vi "log analysis_gps.vi"() -> ()   [LabVIEW 2019] (continued)
-2.475798603,298.940458629,0.4409,0.2946,0.5535,0.1135,0.0926,0.0773,0.0981,0.1029,4.8962,0f000001,0*a1f88c2d\n\t", "INSPVAXA,USB3,0,45.5,FINESTEERING,2107,282909.600,02000000,471d,15824;INS_ALIGNMENT_COMPLETE,INS_RTKFIXED,37.37090578020,126.72380341402,9.0005,22.3000,0.2042,-0.2452,-0.0267,-0.096054371,-2.657817318,299.053399996,0.4409,0.2946,0.5535,0.1135,0.0926,0.0773,0.0981,0.1029,4.8962,0f000001,0*97d4220e\n\t", "INSPVAXA,USB3,0,44.5,FINESTEERING,2107,282910.100,02000000,471d,15824;INS_ALIGNMENT_COMPLETE,INS_RTKFIXED,37.37090649384,126.72380213526,8.9945,22.3000,0.1796,-0.2032,-0.0123,-0.081156055,-2.596786574,299.082136119,0.4412,0.2947,0.5535,0.1135,0.0926,0.0773,0.0981,0.1029,4.8970,0f000001,0*70e9c9df\n\t", "INSPVAXA,USB3,0,44.5,FINESTEERING,2107,282910.600,02000000,471d,15824;INS_ALIGNMENT_COMPLETE,INS_RTKFIXED,37.37090728426,126.72380074897,8.9873,22.3000,0.2078,-0.2346,-0.0218,0.045801771,-2.674891598,299.142927174,0.4412,0.2947,0.5535,0.1135,0.0926,0.0773,0.0981,0.1029,4.8970,0f000001,0*500925c1\n\t", "INSPVAXA,USB3,0,45.5,FINESTEERING,2107,282911.100,02000000,471d,15824;INS_ALIGNMENT_COMPLETE,INS_RTKFIXED,37.37090803309,126.72379945819,8.9800,22.3000,0.1796,-0.1956,-0.0242,0.023894528,-2.705451433,299.250076985,0.4415,0.2948,0.5535,0.1135,0.0925,0.0773,0.0981,0.1029,4.8973,0f000001,0*fcb889be\n\t", "INSPVAXA,USB3,0,45.5,FINESTEERING,2107,282911.600,02000000,471d,15824;INS_ALIGNMENT_COMPLETE,INS_RTKFIXED,37.37090882517,126.72379803977,8.9729,22.3000,0.1992,-0.2347,-0.0122,-0.052701655,-2.537774269,299.314444801,0.4415,0.2948,0.5535,0.1135,0.0925,0.0773,0.0981,0.1029,4.8973,0f000001,0*f806d9f3\n\t", "INSPVAXA,USB3,0,49.0,FINESTEERING,2107,282912.100,02000000,471d,15824;INS_ALIGNMENT_COMPLETE,INS_RTKFIXED,37.37090954144,126.72379680635,8.9662,22.3000,0.2005,-0.2326,-0.0241,-0.125797305,-2.436851943,299.381095140,0.4412,0.2948,0.5534,0.1134,0.0926,0.0773,0.0980,0.1029,4.8978,0f000001,0*e5b9f40a\n\t", "INSPVAXA,USB3,0,49.0,FINESTEERING,2107,282912.600,02000000,471d,15824;INS_ALIGNMENT_COMPLETE,INS_RTKFIXED,37.37091031837,126.72379541279,8.9597,22.3000,0.1852,-0.2068,-0.0204,-0.071142448,-2.486574172,299.492569727,0.4412,0.2948,0.5534,0.1134,0.0926,0.0773,0.0980,0.1029,4.8978,0f000001,0*cac4ba0d\n\t", "INSPVAXA,USB3,0,49.5,FINESTEERING,2107,282913.100,02000000,471d,15824;INS_ALIGNMENT_COMPLETE,INS_RTKFIXED,37.37091108524,126.72379405931,8.9519,22.3000,0.1888,-0.2272,-0.0247,-0.028725670,-2.337365397,299.552597059,0.4407,0.2948,0.5532,0.1133,0.0925,0.0773,0.0980,0.1028,4.8983,0f000001,0*e96bcee1\n\t", "INSPVAXA,USB3,0,49.5,FINESTEERING,2107,282913.600,02000000,471d,15824;INS_ALIGNMENT_COMPLETE,INS_RTKFIXED,37.37091181929,126.72379275953,8.9460,22.3000,0.2010,-0.2341,-0.0266,0.089811982,-2.060196464,299.576677056,0.4407,0.2948,0.5532,0.1133,0.0925,0.0773,0.0980,0.1028,4.8983,0f000001,0*1320fd5f\n\t", "DUALANTENNAHEADINGA,USB3,0,49.5,FINESTEERING,2107,282914.100,02000000,d426,15824;INSUFFICIENT_OBS,NONE,-1.000000000,0.000000000,0.000000000,0.0,0.000000000,0.000000000,\"631T\",13,2,2,2,04,00,20,00*7d7777a8\n\t", "INSPVAXA,USB3,0,52.5,FINESTEERING,2107,282914.600,02000000,471d,15824;INS_ALIGNMENT_COMPLETE,INS_RTKFIXED,37.37091330951,126.72379003668,8.9325,22.3000,0.2030,-0.2221,-0.0237,-0.171357010,-2.043364935,299.558430803,0.4402,0.2946,0.5530,0.1134,0.0925,0.0773,0.0980,0.1028,4.8991,0f000001,0*e9175f83\n\t", "INSPVAXA,USB3,0,50.0,FINESTEERING,2107,282915.100,02000000,471d,15824;INS_ALIGNMENT_COMPLETE,INS_RTKFIXED,37.37091408421,126.72378863973,8.9262,22.3000,0.1969,-0.2337,-0.0140,-0.095383380,-2.265013961,299.603418262,0.4401,0.2946,0.5529,0.1132,0.0924,0.0773,0.0980,0.1028,4.8997,0f000001,0*6f852fd6\n\t", "DUALANTENNAHEADINGA,USB3,0,50.0,FINESTEERING,2107,282915.600,02000000,d426,15824;INSUFFICIENT_OBS,NONE,-1.000000000,0.000000000,0.000000000,0.0,0.000000000,0.000000000,\"631T\",17,2,2,2,04,00,20,00*414acee8\n\t", "DUALANTENNAHEADINGA,USB3,0,48.5,FINESTEERING,2107,282916.100,02000000,d426,15824;INSUFFICIENT_OBS,NONE,-1.000000000,0.000000000,0.000000000,0.0,0.000000000,0.000000000,\"631T\",16,2,2,2,04,00,20,00*fc092504\n\t", "INSPVAXA,USB3,0,48.5,FINESTEERING,2107,282916.600,02000000,471d,15824;INS_ALIGNMENT_COMPLETE,INS_RTKFIXED,37.37091631932,126.72378455605,8.9095,22.3000,0.1948,-0.2448,-0.0204,-0.186363479,-2.427120198,299.446159990,0.4395,0.2945,0.5529,0.1132,0.0924,0.0773,0.0979,0.1028,4.9009,0f000001,0*c1989546\n\t", "INSPVAXA,USB3,0,49.0,FINESTEERING,2107,282917.100,02000000,471d,15824;INS_ALIGNMENT_COMPLETE,INS_RTKFIXED,37.37091707280,126.72378318034,8.9014,22.3000,0.1962,-0.2403,-0.0192,-0.090528151,-2.520576171,299.333268916,0.4392,0.2943,0.5527,0.1132,0.0925,0.0773,0.0979,0.1028,4.9023,0f000001,0*ed058076\n\t", "INSPVAXA,USB3,0,49.0,FINESTEERING,2107,282917.600,02000000,471d,15824;INS_ALIGNMENT_COMPLETE,INS_RTKFIXED,37.37091780195,126.72378182721,8.8930,22.3000,0.1904,-0.2448,-0.0126,-0.105477255,-2.530837408,299.214922397,0.4392,0.2943,0.5527,0.1132,0.0925,0.0773,0.0979,0.1028,4.9023,0f000001,0*48e5530c\n\t", "INSPVAXA,USB3,0,49.5,FINESTEERING,2107,282918.100,02000000,471d,15824;INS_ALIGNMENT_COMPLETE,INS_RTKFIXED,37.37091853728,126.72378045121,8.8866,22.3000,0.1905,-0.2390,-0.0217,-0.320620124,-2.745936216,299.166142272,0.4393,0.2944,0.5528,0.1133,0.0925,0.0773,0.0979,0.1028,4.9038,0f000001,0*f3e51291\n\t", "INSPVAXA,USB3,0,49.5,FINESTEERING,2107,282918.600,02000000,471d,15824;INS_ALIGNMENT_COMPLETE,INS_RTKFIXED,37.37091927039,126.72377907949,8.8817,22.3000,0.1978,-0.2407,-0.0282,-0.339255571,-2.778752767,299.132032456,0.4393,0.2944,0.5528,0.1133,0.0925,0.0773,0.0979,0.1028,4.9038,0f000001,0*ae621dff\n\t", "INSPVAXA,USB3,0,45.0,FINESTEERING,2107,282919.100,02000000,471d,15824;INS_ALIGNMENT_COMPLETE,INS_RTKFIXED,37.37092001431,126.72377771681,8.8758,22.3000,0.1914,-0.2350,-0.0323,-0.346867597,-2.754638155,299.109102683,0.4397,0.2944,0.5532,0.1134,0.0925,0.0773,0.0979,0.1029,4.9053,0f000001,0*63db1984\n\t", "INSPVAXA,USB3,0,45.0,FINESTEERING,2107,282919.600,02000000,471d,15824;INS_ALIGNMENT_COMPLETE,INS_RTKFIXED,37.37092075682,126.72377638763,8.8692,22.3000,0.1933,-0.2372,-0.0282,-0.392529438,-2.688019024,299.098365705,0.4397,0.2944,0.5532,0.1134,0.0925,0.0773,0.0979,0.1029,4.9053,0f000001,0*15ef86f5\n\t", "INSPVAXA,USB3,0,45.0,FINESTEERING,2107,282920.100,02000000,471d,15824;INS_ALIGNMENT_COMPLETE,INS_RTKFIXED,37.37092151983,126.72377503879,8.8627,22.3000,0.1947,-0.2324,-0.0288,-0.374754303,-2.758160229,299.096118379,0.4395,0.2945,0.5534,0.1133,0.0925,0.0773,0.0980,0.1029,4.9066,0f000001,0*6a5bdc77\n\t", "INSPVAXA,USB3,0,50.0,FINESTEERING,2107,282920.600,02000000,471d,15824;INS_ALIGNMENT_COMPLETE,INS_RTKFIXED,37.37092225918,126.72377371320,8.8579,22.3000,0.2080,-0.2433,-0.0263,-0.353123452,-2.702710853,299.168531612,0.4395,0.2945,0.5534,0.1133,0.0925,0.0773,0.0980,0.1029,4.9066,0f000001,0*b7196621\n\t", "DUALANTENNAHEADINGA,USB3,0,50.0,FINESTEERING,2107,282921.100,02000000,d426,15824;INSUFFICIENT_OBS,NONE,-1.000000000,0.000000000,0.000000000,0.0,0.000000000,0.000000000,\"631T\",10,2,2,2,04,00,20,00*711b9acd\n\t", "INSPVAXA,USB3,0,51.0,FINESTEERING,2107,282921.600,02000000,471d,15824;INS_ALIGNMENT_COMPLETE,INS_RTKFIXED,37.37092372084,126.72377106985,8.8494,22.3000,0.2060,-0.2301,-0.0270,-0.435271636,-2.731976151,299.129546059,0.4391,0.2944,0.5533,0.1133,0.0925,0.0773,0.0980,0.1029,4.9078,0f000001,0*5c44fd03\n\t", "DUALANTENNAHEADINGA,USB3,0,51.0,FINESTEERING,2107,282922.100,02000000,d426,15824;INSUFFICIENT_OBS,NONE,-1.000000000,0.000000000,0.000000000,0.0,0.000000000,0.000000000,\"631T\",12,2,2,2,04,00,20,00*d78347f3\n\t", "INSPVAXA,USB3,0,51.0,FINESTEERING,2107,282922.600,02000000,471d,15824;INS_ALIGNMENT_COMPLETE,INS_RTKFIXED,37.37092515994,126.72376843182,8.8389,22.3000,0.2111,-0.2302,-0.0297,-0.438503525,-2.449777885,299.109289893,0.4389,0.2944,0.5534,0.1132,0.0925,0.0773,0.0980,0.1029,4.9089,0f000001,0*6200cf77\n\t", "DUALANTENNAHEADINGA,USB3,0,50.0,FINESTEERING,2107,282923.100,02000000,d426,15824;INSUFFICIENT_OBS,NONE,-1.000000000,0.000000000,0.000000000,0.0,0.000000000,0.000000000,\"631T\",13,2,2,2,04,00,20,00*09fd15d6\n\t", "INSPVAXA,USB3,0,50.0,FINESTEERING,2107,282923.600,02000000,471d,15824;INS_ALIGNMENT_COMPLETE,INS_RTKFIXED,37.37092659742,126.72376579558,8.8280,22.3000,0.2079,-0.2335,-0.0340,-0.348522367,-2.471236219,299.076821205,0.4391,0.2944,0.5534,0.1132,0.0924,0.0773,0.0980,0.1029,4.9102,0f000001,0*b1b4b9cc\n\t", "DUALANTENNAHEADINGA,USB3,0,50.0,FINESTEERING,2107,282924.100,02000000,d426,15824;INSUFFICIENT_OBS,NONE,-1.000000000,0.000000000,0.000000000,0.0,0.000000000,0.000000000,\"631T\",13,2,2,2,04,00,20,00*d3840d98\n\t", "DUALANTENNAHEADINGA,USB3,0,51.0,FINESTEERING,2107,282924.600,02000000,d426,15824;INSUFFICIENT_OBS,NONE,-1.000000000,0.000000000,0.000000000,0.0,0.000000000,0.000000000,\"631T\",13,2,2,2,04,00,20,00*7b68c1aa\n\t", "INSPVAXA,USB3,0,51.5,FINESTEERING,2107,282925.100,02008000,471d,15824;INS_ALIGNMENT_COMPLETE,INS_RTKFIXED,37.37092873619,126.72376179523,8.8090,22.3000,0.2069,-0.2351,-0.0215,-0.632285534,-2.693701140,299.016215129,0.4401,0.2945,0.5538,0.1133,0.0925,0.0773,0.0980,0.1029,4.9131,0f000001,0*70f1efa8\n\t", "DUALANTENNAHEADINGA,USB3,0,51.5,FINESTEERING,2107,282925.600,02008000,d426,15824;INSUFFICIENT_OBS,NONE,-1.000000000,0.000000000,0.000000000,0.0,0.000000000,0.000000000,\"631T\",13,2,2,2,04,00,20,00*5559a71e\n\t", "DUALANTENNAHEADINGA,USB3,0,49.5,FINESTEERING,2107,282926.100,02008000,d426,15824;INSUFFICIENT_OBS,NONE,-1.000000000,0.000000000,0.000000000,0.0,0.000000000,0.000000000,\"631T\",14,2,2,2,04,00,20,00*20bca12d\n\t", "INSPVAXA,USB3,0,49.5,FINESTEERING,2107,282926.600,02008000,471d,15824;INS_ALIGNMENT_COMPLETE,INS_RTKFIXED,37.37093087426,126.72375780222,8.7912,22.3000,0.1944,-0.2057,-0.0172,-0.594741301,-2.946216927,299.056064983,0.4402,0.2946,0.5539,0.1133,0.0925,0.0773,0.0980,0.1029,4.9147,0f000001,0*64625386\n\t", "DUALANTENNAHEADINGA,USB3,0,49.5,FINESTEERING,2107,282927.100,02008000,d426,15824;INSUFFICIENT_OBS,NONE,-1.000000000,0.000000000,0.000000000,0.0,0.000000000,0.000000000,\"631T\",13,2,2,2,04,00,20,00*075a2ebf\n\t", "INSPVAXA,USB3,0,51.0,FINESTEERING,2107,282927.600,02008000,471d,15824;INS_ALIGNMENT_COMPLETE,INS_RTKFIXED,37.37093229253,126.72375516206,8.7796,22.3000,0.1993,-0.2243,-0.0299,-0.537857110,-2.700770606,299.153411685,0.4404,0.2947,0.5542,0.1133,0.0925,0.0773,0.0980,0.1029,4.9162,0f000001,0*499bd090\n\t", "DUALANTENNAHEADINGA,USB3,0,47.5,FINESTEERING,2107,282928.100,02008000,d426,15824;INSUFFICIENT_OBS,NONE,-1.000000000,0.000000000,0.000000000,0.0,0.000000000,0.000000000,\"631T\",16,2,2,2,04,00,20,00*2da4d93a\n\t", "DUALANTENNAHEADINGA,USB3,0,47.5,FINESTEERING,2107,282928.600,02008000,d426,15824;INSUFFICIENT_OBS,NONE,-1.000000000,0.000000000,0.000000000,0.0,0.000000000,0.000000000,\"631T\",16,2,2,2,04,00,20,00*e10cc3ac\n\t", "INSPVAXA,USB3,0,50.5,FINESTEERING,2107,282929.100,02000000,471d,15824;INS_ALIGNMENT_COMPLETE,INS_RTKFIXED,37.37093438604,126.72375124490,8.7687,22.3000,0.1833,-0.2092,-0.0183,-0.594311335,-2.195857139,299.176557510,0.4400,0.2947,0.5540,0.1135,0.0926,0.0773,0.0980,0.1029,4.9192,0f000001,0*a006802b\n\t", "INSPVAXA,USB3,0,50.5,FINESTEERING,2107,282929.600,02000000,471d,15824;INS_ALIGNMENT_COMPLETE,INS_RTKFIXED,37.37093510970,126.72374990284,8.7644,22.3000,0.1889,-0.2243,-0.0171,-0.596042414,-2.165494798,299.266591989,0.4400,0.2947,0.5540,0.1135,0.0926,0.0773,0.0980,0.1029,4.9192,0f000001,0*8915186d\n\t", "INSPVAXA,USB3,0,50.5,FINESTEERING,2107,282930.100,02000000,471d,15824;INS_ALIGNMENT_COMPLETE,INS_RTKFIXED,37.37093581213,126.72374860624,8.7606,22.3000,0.1874,-0.2417,-0.0230,-0.681633205,-2.126475016,299.327076176,0.4420,0.2949,0.5548,0.1137,0.0926,0.0774,0.0980,0.1030,4.9200,0f000001,0*554adfff\n\t", "INSPVAXA,USB3,0,50.5,FINESTEERING,2107,282930.600,02000000,471d,15824;INS_ALIGNMENT_COMPLETE,INS_RTKFIXED,37.37093652868,126.72374728704,8.7566,22.3000,0.1904,-0.2264,-0.0187,-0.696438502,-2.244688797,299.406875205,0.4420,0.2949,0.5548,0.1137,0.0926,0.0774,0.0980,0.1030,4.9200,0f000001,0*0f06850a\n\t", "INSPVAXA,USB3,0,49.0,FINESTEERING,2107,282931.100,02000000,471d,15824;INS_ALIGNMENT_COMPLETE,INS_RTKFIXED,37.37093725237,126.72374594459,8.7526,22.3000,0.1776,-0.2170,-0.0174,-0.804539689,-2.256880287,299.491387164,0.4432,0.2951,0.5553,0.1137,0.0927,0.0774,0.0980,0.1030,4.9204,0f000001,0*08565520\n\t", "DUALANTENNAHEADINGA,USB3,0,49.0,FINESTEERING,2107,282931.600,02000000,d426,15824;INSUFFICIENT_OBS,NONE,-1.000000000,0.000000000,0.000000000,0.0,0.000000000,0.000000000,\"631T\",13,2,2,2,04,00,20,00*c0d8f8a7\n\t", "INSPVAXA,USB3,0,49.0,FINESTEERING,2107,282932.100,02000000,471d,15824;INS_ALIGNMENT_COMPLETE,INS_RTKFIXED,37.37093868529,126.72374334447,8.7450,22.3000,0.1876,-0.2264,-0.0189,-0.905927462,-2.146782726,299.477190532,0.4440,0.2953,0.5559,0.1139,0.0929,0.0774,0.0979,0.1030,4.9203,0f000001,0*aa1aa6b5\n\t", "DUALANTENNAHEADINGA,USB3,0,51.0,FINESTEERING,2107,282932.600,02000000,d426,15824;INSUFFICIENT_OBS,NONE,-1.000000000,0.000000000,0.000000000,0.0,0.000000000,0.000000000,\"631T\",15,2,2,2,04,00,20,00*ae77645a\n\t", "DUALANTENNAHEADINGA,USB3,0,46.0,FINESTEERING,2107,282933.100,02000000,d426,15824;INSUFFICIENT_OBS,NONE,-1.000000000,0.000000000,0.000000000,0.0,0.000000000,0.000000000,\"631T\",15,2,2,2,04,00,20,00*38777e0f\n\t", "DUALANTENNAHEADINGA,USB3,0,46.0,FINESTEERING,2107,282933.600,02000000,d426,15824;INSUFFICIENT_OBS,NONE,-1.000000000,0.000000000,0.000000000,0.0,0.000000000,0.000000000,\"631T\",14,2,2,2,04,00,20,00*233de4c1\n\t", "DUALANTENNAHEADINGA,USB3,0,46.0,FINESTEERING,2107,282934.100,02000000,d426,15824;INSUFFICIENT_OBS,NONE,-1.000000000,0.000000000,0.000000000,0.0,0.000000000,0.000000000,\"631T\",15,2,2,2,04,00,20,00*e20e6641\n\t", "DUALANTENNAHEADINGA,USB3,0,47.5,FINESTEERING,2107,282934.600,02000000,d426,15824;INSUFFICIENT_OBS,NONE,-1.000000000,0.000000000,0.000000000,0.0,0.000000000,0.000000000,\"631T\",17,2,2,2,04,00,20,00*6b2c4a4e\n\t", "DUALANTENNAHEADINGA,USB3,0,47.5,FINESTEERING,2107,282935.100,02000000,d426,15824;INSUFFICIENT_OBS,NONE,-1.000000000,0.000000000,0.000000000,0.0,0.000000000,0.000000000,\"631T\",15,2,2,2,04,00,20,00*bee852f0\n\t", "DUALANTENNAHEADINGA,USB3,0,49.5,FINESTEERING,2107,282935.600,02000000,d426,15824;INSUFFICIENT_OBS,NONE,-1.000000000,0.000000000,0.000000000,0.0,0.000000000,0.000000000,\"631T\",15,2,2,2,04,00,20,00*646f005d\n\t", "DUALANTENNAHEADINGA,USB3,0,49.5,FINESTEERING,2107,282936.100,02000000,d426,15824;INSUFFICIENT_OBS,NONE,-1.000000000,0.000000000,0.000000000,0.0,0.000000000,0.000000000,\"631T\",15,2,2,2,04,00,20,00*1eaf17a0\n\t", "DUALANTENNAHEADINGA,USB3,0,49.5,FINESTEERING,2107,282936.600,02000000,d426,15824;INSUFFICIENT_OBS,NONE,-1.000000000,0.000000000,0.000000000,0.0,0.000000000,0.000000000,\"631T\",15,2,2,2,04,00,20,00*d2070d36\n\t", "DUALANTENNAHEADINGA,USB3,0,49.5,FINESTEERING,2107,282937.100,02000000,d426,15824;INSUFFICIENT_OBS,NONE,-1.000000000,0.000000000,0.000000000,0.0,0.000000000,0.000000000,\"631T\",15,2,2,2,04,00,20,00*73771379\n\t", "DUALANTENNAHEADINGA,USB3,0,50.0,FINESTEERING,2107,282937.600,02000000,d426,15824;INSUFFICIENT_OBS,NONE,-1.000000000,0.000000000,0.000000000,0.0,0.000000000,0.000000000,\"631T\",16,2,2,2,04,00,20,00*68ac25ab\n\t", "DUALANTENNAHEADINGA,USB3,0,50.0,FINESTEERING,2107,282938.100,02000000,d426,15824;INSUFFICIENT_OBS,NONE,-1.000000000,0.000000000,0.000000000,0.0,0.000000000,0.000000000,\"631T\",16,2,2,2,04,00,20,00*a65f0d39\n\t", "DUALANTENNAHEADINGA,USB3,0,50.0,FINESTEERING,2107,282938.600,02000000,d426,15824;INSUFFICIENT_OBS,NONE,-1.000000000,0.000000000,0.000000000,0.0,0.000000000,0.000000000,\"631T\",17,2,2,2,04,00,20,00*bd1597f7\n\t", "DUALANTENNAHEADINGA,USB3,0,50.0,FINESTEERING,2107,282939.100,02000000,d426,15824;INSUFFICIENT_OBS,NONE,-1.000000000,0.000000000,0.000000000,0.0,0.000000000,0.000000000,\"631T\",17,2,2,2,04,00,20,00*1c6589b8\n\t", "DUALANTENNAHEADINGA,USB3,0,52.0,FINESTEERING,2107,282939.600,02000000,d426,15824;INSUFFICIENT_OBS,NONE,-1.000000000,0.000000000,0.000000000,0.0,0.000000000,0.000000000,\"631T\",14,2,2,2,04,00,20,00*bb12b8cf\n\t", "DUALANTENNAHEADINGA,USB3,0,50.0,FINESTEERING,2107,282940.100,02000000,d426,15824;INSUFFICIENT_OBS,NONE,-1.000000000,0.000000000,0.000000000,0.0,0.000000000,0.000000000,\"631T\",14,2,2,2,04,00,20,00*9b77340d\n\t", "INSPVAXA,USB3,0,50.0,FINESTEERING,2107,282940.600,02000000,471d,15824;INS_ALIGNMENT_COMPLETE,INS_RTKFIXED,37.37095109367,126.72372052515,8.6731,22.3000,0.1517,-0.2300,-0.0234,-0.267173329,-2.329530247,298.720230899,0.4406,0.2945,0.5541,0.1133,0.0925,0.0773,0.0978,0.1028,4.9197,0f000001,0*f2292127\n\t", "DUALANTENNAHEADINGA,USB3,0,49.5,FINESTEERING,2107,282941.100,02000000,d426,15824;INSUFFICIENT_OBS,NONE,-1.000000000,0.000000000,0.000000000,0.0,0.000000000,0.000000000,\"631T\",17,2,2,2,04,00,20,00*21dc1c90\n\t", "DUALANTENNAHEADINGA,USB3,0,49.5,FINESTEERING,2107,282941.600,02000000,d426,15824;INSUFFICIENT_OBS,NONE,-1.000000000,0.000000000,0.000000000,0.0,0.000000000,0.000000000,\"631T\",17,2,2,2,04,00,20,00*ed740606\n\t", "DUALANTENNAHEADINGA,USB3,0,49.5,FINESTEERING,2107,282942.100,02000000,d426,15824;INSUFFICIENT_OBS,NONE,-1.000000000,0.000000000,0.000000000,0.0,0.000000000,0.000000000,\"631T\",15,2,2,2,04,00,20,00*e300170a\n\t", "DUALANTENNAHEADINGA,USB3,0,49.5,FINESTEERING,2107,282942.600,02000000,d426,15824;INSUFFICIENT_OBS,NONE,-1.000000000,0.000000000,0.000000000,0.0,0.000000000,0.000000000,\"631T\",13,2,2,2,04,00,20,00*b274068f\n\t", "DUALANTENNAHEADINGA,USB3,0,49.5,FINESTEERING,2107,282943.100,02008000,d426,15824;INSUFFICIENT_OBS,NONE,-1.000000000,0.000000000,0.000000000,0.0,0.000000000,0.000000000,\"631T\",13,2,2,2,04,00,20,00*05979c61\n\t", "DUALANTENNAHEADINGA,USB3,0,50.0,FINESTEERING,2107,282943.600,02008000,d426,15824;INSUFFICIENT_OBS,NONE,-1.000000000,0.000000000,0.000000000,0.0,0.000000000,0.000000000,\"631T\",15,2,2,2,04,00,20,00*20c62709\n\t", "DUALANTENNAHEADINGA,USB3,0,50.0,FINESTEERING,2107,282944.100,02008000,d426,15824;INSUFFICIENT_OBS,NONE,-1.000000000,0.000000000,0.000000000,0.0,0.000000000,0.000000000,\"631T\",15,2,2,2,04,00,20,00*361725d1\n\t", "DUALANTENNAHEADINGA,USB3,0,53.0,FINESTEERING,2107,282944.600,02008000,d426,15824;INSUFFICIENT_OBS,NONE,-1.000000000,0.000000000,0.000000000,0.0,0.000000000,0.000000000,\"631T\",15,2,2,2,04,00,20,00*567244ab\n\t", "DUALANTENNAHEADINGA,USB3,0,52.5,FINESTEERING,2107,282945.100,02008000,d426,15824;INSUFFICIENT_OBS,NONE,-1.000000000,0.000000000,0.000000000,0.0,0.000000000,0.000000000,\"631T\",13,2,2,2,04,00,20,00*5be0619f\n\t", "DUALANTENNAHEADINGA,USB3,0,52.5,FINESTEERING,2107,282945.600,02008000,d426,15824;INSUFFICIENT_OBS,NONE,-1.000000000,0.000000000,0.000000000,0.0,0.000000000,0.000000000,\"631T\",13,2,2,2,04,00,20,00*97487b09\n\t", "DUALANTENNAHEADINGA,USB3,0,49.5,FINESTEERING,2107,282946.100,02008000,d426,15824;INSUFFICIENT_OBS,NONE,-1.000000000,0.000000000,0.000000000,0.0,0.000000000,0.000000000,\"631T\",14,2,2,2,04,00,20,00*4e6006d6\n\t", "DUALANTENNAHEADINGA,USB3,0,49.5,FINESTEERING,2107,282946.600,02008000,d426,15824;INSUFFICIENT_OBS,NONE,-1.000000000,0.000000000,0.000000000,0.0,0.000000000,0.000000000,\"631T\",15,2,2,2,04,00,20,00*552a9c18\n\t", "DUALANTENNAHEADINGA,USB3,0,48.5,FINESTEERING,2107,282947.100,02008000,d426,15824;INSUFFICIENT_OBS,NONE,-1.000000000,0.000000000,0.000000000,0.0,0.000000000,0.000000000,\"631T\",16,2,2,2,04,00,20,00*3348d25a\n\t", "DUALANTENNAHEADINGA,USB3,0,48.5,FINESTEERING,2107,282947.600,02000000,d426,15824;INSUFFICIENT_OBS,NONE,-1.000000000,0.000000000,0.000000000,0.0,0.000000000,0.000000000,\"631T\",16,2,2,2,04,00,20,00*e9734c6d\n\t", "DUALANTENNAHEADINGA,USB3,0,48.5,FINESTEERING,2107,282948.100,02000000,d426,15824;INSUFFICIENT_OBS,NONE,-1.000000000,0.000000000,0.000000000,0.0,0.000000000,0.000000000,\"631T\",16,2,2,2,04,00,20,00*278064ff\n\t", "DUALANTENNAHEADINGA,USB3,0,49.0,FINESTEERING,2107,282948.600,02000000,d426,15824;INSUFFICIENT_OBS,NONE,-1.000000000,0.000000000,0.000000000,0.0,0.000000000,0.000000000,\"631T\",16,2,2,2,04,00,20,00*da164e01\n\t", "DUALANTENNAHEADINGA,USB3,0,49.0,FINESTEERING,2107,282949.100,02008000,d426,15824;INSUFFICIENT_OBS,NONE,-1.000000000,0.000000000,0.000000000,0.0,0.000000000,0.000000000,\"631T\",16,2,2,2,04,00,20,00*6df5d4ef\n\t", "DUALANTENNAHEADINGA,USB3,0,50.5,FINESTEERING,2107,282949.600,02008000,d426,15824;INSUFFICIENT_OBS,NONE,-1.000000000,0.000000000,0.000000000,0.0,0.000000000,0.000000000,\"631T\",16,2,2,2,04,00,20,00*d5786494\n\t", "DUALANTENNAHEADINGA,USB3,0,50.5,FINESTEERING,2107,282950.100,02008000,d426,15824;INSUFFICIENT_OBS,NONE,-1.000000000,0.000000000,0.000000000,0.0,0.000000000,0.000000000,\"631T\",16,2,2,2,04,00,20,00*5348e2e5\n\t", "DUALANTENNAHEADINGA,USB3,0,50.5,FINESTEERING,2107,282950.600,02008000,d426,15824;INSUFFICIENT_OBS,NONE,-1.000000000,0.000000000,0.000000000,0.0,0.000000000,0.000000000,\"631T\",16,2,2,2,04,00,20,00*9fe0f873\n\t", "DUALANTENNAHEADINGA,USB3,0,48.0,FINESTEERING,2107,282951.100,02008000,d426,15824;INSUFFICIENT_OBS,NONE,-1.000000000,0.000000000,0.000000000,0.0,0.000000000,0.000000000,\"631T\",16,2,2,2,04,00,20,00*2ef19a75\n\t", "DUALANTENNAHEADINGA,USB3,0,48.0,FINESTEERING,2107,282951.600,02008000,d426,15824;INSUFFICIENT_OBS,NONE,-1.000000000,0.000000000,0.000000000,0.0,0.000000000,0.000000000,\"631T\",17,2,2,2,04,00,20,00*35bb00bb\n\t", "DUALANTENNAHEADINGA,USB3,0,47.5,FINESTEERING,2107,282953.100,02008000,d426,15824;INSUFFICIENT_OBS,NONE,-1.000000000,0.000000000,0.000000000,0.0,0.000000000,0.000000000,\"631T\",14,2,2,2,04,00,20,00*a6e4ed65\n\t", "DUALANTENNAHEADINGA,USB3,0,50.0,FINESTEERING,2107,282953.600,02000000,d426,15824;INSUFFICIENT_OBS,NONE,-1.000000000,0.000000000,0.000000000,0.0,0.000000000,0.000000000,\"631T\",13,2,2,2,04,00,20,00*54eb1acf\n\t", "DUALANTENNAHEADINGA,USB3,0,48.0,FINESTEERING,2107,282954.100,02000000,d426,15824;INSUFFICIENT_OBS,NONE,-1.000000000,0.000000000,0.000000000,0.0,0.000000000,0.000000000,\"631T\",14,2,2,2,04,00,20,00*4d1f09d9\n\t", "DUALANTENNAHEADINGA,USB3,0,48.0,FINESTEERING,2107,282954.600,02000000,d426,15824;INSUFFICIENT_OBS,NONE,-1.000000000,0.000000000,0.000000000,0.0,0.000000000,0.000000000,\"631T\",16,2,2,2,04,00,20,00*f50315be\n\t", "INSPVAXA,USB3,0,47.5,FINESTEERING,2107,282955.150,02000000,471d,15824;INS_ALIGNMENT_COMPLETE,INS_RTKFIXED,37.37097191028,126.72368135449,8.4841,22.3000,0.1693,-0.2422,-0.0142,-0.799407397,-2.166438439,297.747094152,0.4450,0.2953,0.5584,0.1141,0.0928,0.0775,0.0978,0.1030,4.9299,0f000001,0*711ec271\n\t", "DUALANTENNAHEADINGA,USB3,0,47.5,FINESTEERING,2107,282955.600,02000000,d426,15824;INSUFFICIENT_OBS,NONE,-1.000000000,0.000000000,0.000000000,0.0,0.000000000,0.000000000,\"631T\",13,2,2,2,04,00,20,00*8140e48e\n\t", "DUALANTENNAHEADINGA,USB3,0,47.5,FINESTEERING,2107,282956.100,02000000,d426,15824;INSUFFICIENT_OBS,NONE,-1.000000000,0.000000000,0.000000000,0.0,0.000000000,0.000000000,\"631T\",14,2,2,2,04,00,20,00*b1be7838\n\t", "DUALANTENNAHEADINGA,USB3,0,49.5,FINESTEERING,2107,282957.100,02000000,d426,15824;INSUFFICIENT_OBS,NONE,-1.000000000,0.000000000,0.000000000,0.0,0.000000000,0.000000000,\"631T\",15,2,2,2,04,00,20,00*1dabb482\n\t", "DUALANTENNAHEADINGA,USB3,0,47.5,FINESTEERING,2107,282958.100,02000000,d426,15824;INSUFFICIENT_OBS,NONE,-1.000000000,0.000000000,0.000000000,0.0,0.000000000,0.000000000,\"631T\",14,2,2,2,04,00,20,00*de3d4ee5\n\t", "DUALANTENNAHEADINGA,USB3,0,47.5,FINESTEERING,2107,282958.600,02000000,d426,15824;INSUFFICIENT_OBS,NONE,-1.000000000,0.000000000,0.000000000,0.0,0.000000000,0.000000000,\"631T\",15,2,2,2,04,00,20,00*c577d42b\n\t", "DUALANTENNAHEADINGA,USB3,0,47.5,FINESTEERING,2107,282959.100,02000000,d426,15824;INSUFFICIENT_OBS,NONE,-1.000000000,0.000000000,0.000000000,0.0,0.000000000,0.000000000,\"631T\",15,2,2,2,04,00,20,00*6407ca64\n\t", "INSPVAXA,USB3,0,50.5,FINESTEERING,2107,282959.650,02000000,471d,15824;INS_ALIGNMENT_COMPLETE,INS_RTKFIXED,37.37097835365,126.72366921356,8.4679,22.3000,0.1677,-0.2288,-0.0117,-1.228660842,-1.304176220,297.349897082,0.4459,0.2954,0.5577,0.1140,0.0926,0.0775,0.0977,0.1029,4.9210,0f000001,0*0060fe10\n\t", "DUALANTENNAHEADINGA,USB3,0,50.5,FINESTEERING,2107,282960.100,02000000,d426,15824;INSUFFICIENT_OBS,NONE,-1.000000000,0.000000000,0.000000000,0.0,0.000000000,0.000000000,\"631T\",15,2,2,2,04,00,20,00*3c5b3030\n\t", "INSPVAXA,USB3,0,51.0,FINESTEERING,2107,282960.650,02000000,471d,15824;INS_ALIGNMENT_COMPLETE,INS_RTKFIXED,37.37097975694,126.72366653039,8.4696,22.3000,0.1798,-0.2500,-0.0237,-1.216813697,-1.020291327,297.186745647,0.4456,0.2953,0.5575,0.1139,0.0925,0.0775,0.0977,0.1029,4.9186,0f000001,0*5a2daee3\n\t", "INSPVAXA,USB3,0,49.5,FINESTEERING,2107,282961.150,02000000,471d,15824;INS_ALIGNMENT_COMPLETE,INS_RTKFIXED,37.37098043030,126.72366522949,8.4707,22.3000,0.1736,-0.2321,-0.0202,-1.283284978,-0.599057557,297.054686065,0.4445,0.2952,0.5571,0.1143,0.0927,0.0774,0.0977,0.1029,4.9180,0f000001,0*2a0011a7\n\t", "INSPVAXA,USB3,0,49.5,FINESTEERING,2107,282961.650,02000000,471d,15824;INS_ALIGNMENT_COMPLETE,INS_RTKFIXED,37.37098110598,126.72366388035,8.4719,22.3000,0.1770,-0.2280,-0.0121,-1.256734813,-0.468526874,296.976116975,0.4445,0.2952,0.5571,0.1143,0.0927,0.0774,0.0977,0.1029,4.9180,0f000001,0*1df4362b\n\t", "INSPVAXA,USB3,0,47.5,FINESTEERING,2107,282962.650,02000000,471d,15824;INS_ALIGNMENT_COMPLETE,INS_RTKFIXED,37.37098248042,126.72366115831,8.4743,22.3000,0.1748,-0.2259,-0.0058,-1.109471355,-0.449070026,296.783460113,0.4449,0.2952,0.5570,0.1145,0.0926,0.0774,0.0977,0.1028,4.9165,0f000001,0*1baf4086\n\t", "INSPVAXA,USB3,0,50.0,FINESTEERING,2107,282963.150,02000000,471d,15824;INS_ALIGNMENT_COMPLETE,INS_RTKFIXED,37.37098316293,126.72365977185,8.4754,22.3000,0.1768,-0.2291,-0.0058,-1.166384904,-0.522599748,296.670399904,0.4455,0.2951,0.5568,0.1141,0.0925,0.0774,0.0977,0.1028,4.9146,0f000001,0*0f185e23\n\t", "INSPVAXA,USB3,0,50.0,FINESTEERING,2107,282963.650,02000000,471d,15824;INS_ALIGNMENT_COMPLETE,INS_RTKFIXED,37.37098384842,126.72365839732,8.4765,22.3000,0.1700,-0.2283,-0.0073,-1.035044239,-0.558854853,296.631402056,0.4455,0.2951,0.5568,0.1141,0.0925,0.0774,0.0977,0.1028,4.9146,0f000001,0*d0797a7e\n\t", "INSPVAXA,USB3,0,47.5,FINESTEERING,2107,282964.150,02000000,471d,15824;INS_ALIGNMENT_COMPLETE,INS_RTKFIXED,37.37098452995,126.72365703977,8.4774,22.3000,0.1687,-0.2278,-0.0051,-0.825749574,-0.403704202,296.577547873,0.4447,0.2949,0.5563,0.1141,0.0926,0.0774,0.0977,0.1028,4.9134,0f000001,0*96a6dd12\n\t", "DUALANTENNAHEADINGA,USB3,0,47.5,FINESTEERING,2107,282964.600,02000000,d426,15824;INSUFFICIENT_OBS,NONE,-1.000000000,0.000000000,0.000000000,0.0,0.000000000,0.000000000,\"631T\",13,2,2,2,04,00,20,00*364e308a\n\t", "INSPVAXA,USB3,0,49.0,FINESTEERING,2107,282965.150,02000000,471d,15824;INS_ALIGNMENT_COMPLETE,INS_RTKFIXED,37.37098586278,126.72365430292,8.4776,22.3000,0.1652,-0.2280,-0.0084,-0.812912729,-0.298745474,296.545314243,0.4441,0.2948,0.5560,0.1139,0.0926,0.0774,0.0977,0.1027,4.9127,0f000001,0*10118c42\n\t", "INSPVAXA,USB3,0,49.0,FINESTEERING,2107,282965.650,02000000,471d,15824;INS_ALIGNMENT_COMPLETE,INS_RTKFIXED,37.37098653582,126.72365294600,8.4789,22.3000,0.1677,-0.2410,-0.0069,-0.826772315,0.019774028,296.533621438,0.4441,0.2948,0.5560,0.1139,0.0926,0.0774,0.0977,0.1027,4.9127,0f000001,0*1d42ccbf\n\t", "DUALANTENNAHEADINGA,USB3,0,48.5,FINESTEERING,2107,282967.100,02000000,d426,15824;INSUFFICIENT_OBS,NONE,-1.000000000,0.000000000,0.000000000,0.0,0.000000000,0.000000000,\"631T\",13,2,2,2,04,00,20,00*3ee5b9e8\n\t", "INSPVAXA,USB3,0,48.5,FINESTEERING,2107,282967.650,02000000,471d,15824;INS_ALIGNMENT_COMPLETE,INS_RTKFIXED,37.37098925178,126.72364742874,8.4811,22.3000,0.1700,-0.2499,-0.0176,-0.986615151,-0.569191402,296.569428788,0.4450,0.2948,0.5562,0.1138,0.0925,0.0774,0.0977,0.1027,4.9114,0f000001,0*8120b203\n\t", "INSPVAXA,USB3,0,51.0,FINESTEERING,2107,282968.150,02000000,471d,15824;INS_ALIGNMENT_COMPLETE,INS_RTKFIXED,37.37098994015,126.72364604242,8.4821,22.3000,0.1610,-0.2295,-0.0122,-1.022493310,-0.855866678,296.640582701,0.4448,0.2947,0.5563,0.1137,0.0927,0.0774,0.0977,0.1027,4.9112,0f000001,0*d8f4721a\n\t", "INSPVAXA,USB3,0,51.0,FINESTEERING,2107,282968.650,02000000,471d,15824;INS_ALIGNMENT_COMPLETE,INS_RTKFIXED,37.37099061783,126.72364467060,8.4818,22.3000,0.1613,-0.2282,-0.0121,-1.153302728,-0.788505440,296.737399277,0.4448,0.2947,0.5563,0.1137,0.0927,0.0774,0.0977,0.1027,4.9112,0f000001,0*561016f0\n\t", "INSPVAXA,USB3,0,51.0,FINESTEERING,2107,282969.150,02000000,471d,15824;INS_ALIGNMENT_COMPLETE,INS_RTKFIXED,37.37099130336,126.72364331886,8.4815,22.3000,0.1682,-0.2376,-0.0147,-1.125512606,-0.794604526,296.797111789,0.4434,0.2946,0.5560,0.1136,0.0926,0.0774,0.0977,0.1027,4.9114,0f000001,0*989702a1\n\t", "INSPVAXA,USB3,0,51.0,FINESTEERING,2107,282969.650,02000000,471d,15824;INS_ALIGNMENT_COMPLETE,INS_RTKFIXED,37.37099198077,126.72364195097,8.4825,22.3000,0.1618,-0.2351,-0.0139,-1.127841235,-0.916992124,296.845405459,0.4434,0.2946,0.5560,0.1136,0.0926,0.0774,0.0977,0.1027,4.9114,0f000001,0*282a9ea8\n\t", "INSPVAXA,USB3,0,49.5,FINESTEERING,2107,282970.150,02000000,471d,15824;INS_ALIGNMENT_COMPLETE,INS_RTKFIXED,37.37099263807,126.72364060691,8.4830,22.3000,0.1632,-0.2345,-0.0165,-1.327041845,-0.755974067,296.808985126,0.4427,0.2946,0.5559,0.1136,0.0925,0.0774,0.0977,0.1027,4.9120,0f000001,0*fb111f10\n\t", "INSPVAXA,USB3,0,49.5,FINESTEERING,2107,282970.650,02000000,471d,15824;INS_ALIGNMENT_COMPLETE,INS_RTKFIXED,37.37099330542,126.72363923345,8.4843,22.3000,0.1650,-0.2334,-0.0103,-1.379297675,-0.666693531,296.810188523,0.4427,0.2946,0.5559,0.1136,0.0925,0.0774,0.0977,0.1027,4.9120,0f000001,0*40e7d89f\n\t", "INSPVAXA,USB3,0,50.5,FINESTEERING,2107,282971.150,02000000,471d,15824;INS_ALIGNMENT_COMPLETE,INS_RTKFIXED,37.37099398804,126.72363786563,8.4853,22.3000,0.1661,-0.2338,-0.0180,-1.270685032,-0.682780948,296.817282496,0.4423,0.2946,0.5559,0.1136,0.0925,0.0774,0.0977,0.1027,4.9128,0f000001,0*f8a30bce\n\t", "INSPVAXA,USB3,0,50.5,FINESTEERING,2107,282971.650,02000000,471d,15824;INS_ALIGNMENT_COMPLETE,INS_RTKFIXED,37.37099465990,126.72363651456,8.4846,22.3000,0.1699,-0.2362,-0.0068,-1.125018269,-0.570550984,296.760377501,0.4423,0.2946,0.5559,0.1136,0.0925,0.0774,0.0977,0.1027,4.9128,0f000001,0*ee20163a\n\t", "INSPVAXA,USB3,0,48.5,FINESTEERING,2107,282972.150,02000000,471d,15824;INS_ALIGNMENT_COMPLETE,INS_RTKFIXED,37.37099533114,126.72363514569,8.4846,22.3000,0.1631,-0.2434,-0.0075,-1.229353207,-0.492392608,296.737479032,0.4422,0.2946,0.5560,0.1136,0.0925,0.0774,0.0977,0.1027,4.9138,0f000001,0*e2a3fa7c\n\t", "INSPVAXA,USB3,0,48.5,FINESTEERING,2107,282972.650,02000000,471d,15824;INS_ALIGNMENT_COMPLETE,INS_RTKFIXED,37.37099601296,126.72363373726,8.4848,22.3000,0.1655,-0.2434,-0.0062,-1.394785800,-0.542379073,296.812195855,0.4422,0.2946,0.5560,0.1136,0.0925,0.0774,0.0977,0.1027,4.9138,0f000001,0*ee63dd76\n\t", "INSPVAXA,USB3,0,47.0,FINESTEERING,2107,282973.150,02000000,471d,15824;INS_ALIGNMENT_COMPLETE,INS_RTKFIXED,37.37099670386,126.72363233646,8.4846,22.3000,0.1605,-0.2379,-0.0037,-1.521129756,-0.763571260,296.778124874,0.4424,0.2946,0.5561,0.1137,0.0925,0.0774,0.0977,0.1027,4.9150,0f000001,0*6c9cf6ab\n\t", "INSPVAXA,USB3,0,47.0,FINESTEERING,2107,282973.650,02000000,471d,15824;INS_ALIGNMENT_COMPLETE,INS_RTKFIXED,37.37099738989,126.72363093033,8.4852,22.3000,0.1673,-0.2327,0.0049,-1.602600322,-0.872352235,296.775722188,0.4424,0.2946,0.5561,0.1137,0.0925,0.0774,0.0977,0.1027,4.9150,0f000001,0*6d258e45\n\t", "INSPVAXA,USB3,0,49.0,FINESTEERING,2107,282974.650,02000000,471d,15824;INS_ALIGNMENT_COMPLETE,INS_RTKFIXED,37.37099878397,126.72362813918,8.4887,22.3000,0.1782,-0.2307,0.0009,-1.519938045,-1.116202869,296.818721301,0.4416,0.2946,0.5560,0.1136,0.0925,0.0774,0.0977,0.1027,4.9163,0f000001,0*219b4438\n\t", "INSPVAXA,USB3,0,48.5,FINESTEERING,2107,282975.150,02000000,471d,15824;INS_ALIGNMENT_COMPLETE,INS_RTKFIXED,37.37099949137,126.72362674599,8.4896,22.3000,0.1736,-0.2362,0.0047,-1.445494984,-1.113340101,296.818619206,0.4431,0.2948,0.5567,0.1139,0.0926,0.0775,0.0977,0.1028,4.9177,0f000001,0*6f5d7051\n\t", "INSPVAXA,USB3,0,48.5,FINESTEERING,2107,282975.650,02000000,471d,15824;INS_ALIGNMENT_COMPLETE,INS_RTKFIXED,37.37100019826,126.72362538278,8.4881,22.3000,0.1707,-0.2363,0.0005,-1.379938720,-0.916519890,296.842609438,0.4431,0.2948,0.5567,0.1139,0.0926,0.0775,0.0977,0.1028,4.9177,0f000001,0*5514ce87\n\t", "INSPVAXA,USB3,0,49.5,FINESTEERING,2107,282976.150,02000000,471d,15824;INS_ALIGNMENT_COMPLETE,INS_RTKFIXED,37.37100091207,126.72362400101,8.4878,22.3000,0.1676,-0.2422,-0.0038,-1.345011262,-0.792526169,296.841980964,0.4425,0.2947,0.5567,0.1137,0.0926,0.0775,0.0977,0.1027,4.9188,0f000001,0*da02f91b\n\t", "INSPVAXA,USB3,0,49.5,FINESTEERING,2107,282976.650,02000000,471d,15824;INS_ALIGNMENT_COMPLETE,INS_RTKFIXED,37.37100161787,126.72362259542,8.4876,22.3000,0.1713,-0.2361,-0.0000,-1.230290635,-0.956554131,296.705725068,0.4425,0.2947,0.5567,0.1137,0.0926,0.0775,0.0977,0.1027,4.9188,0f000001,0*8e2a3525\n\t", "INSPVAXA,USB3,0,50.0,FINESTEERING,2107,282977.150,02000000,471d,15824;INS_ALIGNMENT_COMPLETE,INS_RTKFIXED,37.37100231261,126.72362121390,8.4877,22.3000,0.1651,-0.2421,0.0008,-1.098832221,-0.904742170,296.548603231,0.4420,0.2947,0.5566,0.1136,0.0926,0.0774,0.0977,0.1027,4.9199,0f000001,0*083bf95e\n\t", "INSPVAXA,USB3,0,50.0,FINESTEERING,2107,282977.650,02000000,471d,15824;INS_ALIGNMENT_COMPLETE,INS_RTKFIXED,37.37100299121,126.72361981257,8.4879,22.3000,0.1659,-0.2302,-0.0060,-1.021895005,-0.933563278,296.461558193,0.4420,0.2947,0.5566,0.1136,0.0926,0.0774,0.0977,0.1027,4.9199,0f000001,0*f0f7e65a\n\t", "INSPVAXA,USB3,0,52.0,FINESTEERING,2107,282978.150,02000000,471d,15824;INS_ALIGNMENT_COMPLETE,INS_RTKFIXED,37.37100367247,126.72361842907,8.4879,22.3000,0.1629,-0.2311,-0.0012,-0.920604944,-1.043526299,296.260165463,0.4427,0.2948,0.5570,0.1137,0.0928,0.0775,0.0977,0.1027,4.9208,0f000001,0*6c36e752\n\t", "INSPVAXA,USB3,0,52.0,FINESTEERING,2107,282978.650,02000000,471d,15824;INS_ALIGNMENT_COMPLETE,INS_RTKFIXED,37.37100436684,126.72361701359,8.4867,22.3000,0.1639,-0.2335,-0.0162,-0.883856990,-1.214783963,296.168399886,0.4427,0.2948,0.5570,0.1137,0.0928,0.0775,0.0977,0.1027,4.9208,0f000001,0*f7bb67d2\n\t", "INSPVAXA,USB3,0,51.5,FINESTEERING,2107,282979.150,02000000,471d,15824;INS_ALIGNMENT_COMPLETE,INS_RTKFIXED,37.37100504962,126.72361562716,8.4847,22.3000,0.1600,-0.2330,-0.0182,-0.879226259,-1.131302419,296.112400832,0.4429,0.2948,0.5572,0.1137,0.0928,0.0775,0.0977,0.1027,4.9212,0f000001,0*44fc000f\n\t", "INSPVAXA,USB3,0,48.0,FINESTEERING,2107,282980.150,02000000,471d,15824;INS_ALIGNMENT_COMPLETE,INS_RTKFIXED,37.37100639827,126.72361280580,8.4843,22.3000,0.1610,-0.2464,-0.0078,-1.128808360,-1.315408116,295.882124797,0.4447,0.2950,0.5582,0.1140,0.0927,0.0775,0.0977,0.1028,4.9213,0f000001,0*5399c86c\n\t", "INSPVAXA,USB3,0,48.0,FINESTEERING,2107,282980.650,02000000,471d,15824;INS_ALIGNMENT_COMPLETE,INS_RTKFIXED,37.37100705164,126.72361137761,8.4834,22.3000,0.1707,-0.2402,-0.0119,-1.407160941,-1.329354223,295.708309677,0.4447,0.2950,0.5582,0.1140,0.0927,0.0775,0.0977,0.1028,4.9213,0f000001,0*d4834280\n\t", "INSPVAXA,USB3,0,48.5,FINESTEERING,2107,282981.150,02000000,471d,15824;INS_ALIGNMENT_COMPLETE,INS_RTKFIXED,37.37100772173,126.72360998460,8.4814,22.3000,0.1860,-0.2371,-0.0157,-1.203417733,-1.261430362,295.578766556,0.4455,0.2951,0.5589,0.1141,0.0926,0.0776,0.0977,0.1028,4.9213,0f000001,0*2091f446\n\t", "INSPVAXA,USB3,0,51.0,FINESTEERING,2107,282983.150,02000000,471d,15824;INS_ALIGNMENT_COMPLETE,INS_RTKFIXED,37.37101036366,126.72360442489,8.4628,22.3000,0.1755,-0.2357,-0.0080,-1.025739547,-1.189368406,295.388361945,0.4463,0.2951,0.5596,0.1141,0.0926,0.0776,0.0978,0.1028,4.9221,0f000001,0*2959208b\n\t", "INSPVAXA,USB3,0,51.0,FINESTEERING,2107,282983.650,02000000,471d,15824;INS_ALIGNMENT_COMPLETE,INS_RTKFIXED,37.37101102324,126.72360304881,8.4600,22.3000,0.1712,-0.2258,-0.0116,-0.859579681,-1.039097489,295.288660935,0.4463,0.2951,0.5596,0.1141,0.0926,0.0776,0.0978,0.1028,4.9221,0f000001,0*ad7af1a9\n\t", "INSPVAXA,USB3,0,50.5,FINESTEERING,2107,282984.150,02008000,471d,15824;INS_ALIGNMENT_COMPLETE,INS_RTKFIXED,37.37101166488,126.72360167491,8.4566,22.3000,0.1754,-0.2281,-0.0207,-0.961299584,-0.781860574,295.230299277,0.4466,0.2950,0.5599,0.1142,0.0925,0.0776,0.0978,0.1028,4.9229,0f000001,0*2cbfc422\n\t", "INSPVAXA,USB3,0,46.0,FINESTEERING,2107,282985.150,02008000,471d,15824;INS_ALIGNMENT_COMPLETE,INS_RTKFIXED,37.37101294073,126.72359895253,8.4524,22.3000,0.1696,-0.2376,-0.0054,-0.854565815,-0.366619104,295.159142315,0.4467,0.2950,0.5599,0.1143,0.0926,0.0776,0.0978,0.1028,4.9242,0f000001,0*a94814eb\n\t", "INSPVAXA,USB3,0,46.0,FINESTEERING,2107,282985.650,02008000,471d,15824;INS_ALIGNMENT_COMPLETE,INS_RTKFIXED,37.37101359136,126.72359755019,8.4503,22.3000,0.1680,-0.2437,-0.0157,-0.803804661,-0.502558693,295.184613052,0.4467,0.2950,0.5599,0.1143,0.0926,0.0776,0.0978,0.1028,4.9242,0f000001,0*db0a5a5c\n\t", "INSPVAXA,USB3,0,46.5,FINESTEERING,2107,282986.150,02008000,471d,15824;INS_ALIGNMENT_COMPLETE,INS_RTKFIXED,37.37101422818,126.72359615090,8.4473,22.3000,0.1631,-0.2437,-0.0170,-1.039180574,-0.597901795,295.266800009,0.4472,0.2951,0.5600,0.1141,0.0926,0.0776,0.0978,0.1028,4.9255,0f000001,0*b918d4c4\n\t", "INSPVAXA,USB3,0,51.5,FINESTEERING,2107,282988.150,02000000,471d,15824;INS_ALIGNMENT_COMPLETE,INS_RTKFIXED,37.37101680407,126.72359058877,8.4432,22.3000,0.1712,-0.2477,-0.0072,-1.132987341,-0.795555306,295.241601401,0.4472,0.2951,0.5599,0.1141,0.0926,0.0776,0.0978,0.1028,4.9272,0f000001,0*1b3b971d\n\t", "INSPVAXA,USB3,0,51.5,FINESTEERING,2107,282988.650,02000000,471d,15824;INS_ALIGNMENT_COMPLETE,INS_RTKFIXED,37.37101744623,126.72358920504,8.4402,22.3000,0.1681,-0.2455,-0.0077,-0.918184944,-0.964879494,295.259837239,0.4472,0.2951,0.5599,0.1141,0.0926,0.0776,0.0978,0.1028,4.9272,0f000001,0*72c9ff23\n\t", "INSPVAXA,USB3,0,52.0,FINESTEERING,2107,282989.150,02000000,471d,15824;INS_ALIGNMENT_COMPLETE,INS_RTKFIXED,37.37101810010,126.72358780342,8.4378,22.3000,0.1635,-0.2346,-0.0127,-0.821579606,-1.181208357,295.261813725,0.4470,0.2950,0.5598,0.1141,0.0925,0.0776,0.0977,0.1028,4.9279,0f000001,0*084187d8\n\t", "INSPVAXA,USB3,0,52.0,FINESTEERING,2107,282989.650,02000000,471d,15824;INS_ALIGNMENT_COMPLETE,INS_RTKFIXED,37.37101876823,126.72358639475,8.4359,22.3000,0.1596,-0.2371,-0.0062,-0.715677130,-1.181942284,295.239523711,0.4470,0.2950,0.5598,0.1141,0.0925,0.0776,0.0977,0.1028,4.9279,0f000001,0*db6d0e7d\n\t", "INSPVAXA,USB3,0,50.0,FINESTEERING,2107,282990.150,02000000,471d,15824;INS_ALIGNMENT_COMPLETE,INS_RTKFIXED,37.37101943584,126.72358497714,8.4335,22.3000,0.1613,-0.2440,-0.0113,-0.746627018,-1.102743180,295.224075586,0.4466,0.2950,0.5597,0.1141,0.0925,0.0776,0.0977,0.1028,4.9289,0f000001,0*6b0a1647\n\t", "INSPVAXA,USB3,0,50.0,FINESTEERING,2107,282990.650,02000000,471d,15824;INS_ALIGNMENT_COMPLETE,INS_RTKFIXED,37.37102009853,126.72358357998,8.4311,22.3000,0.1630,-0.2513,-0.0092,-0.640841059,-0.917447835,295.078324917,0.4466,0.2950,0.5597,0.1141,0.0925,0.0776,0.0977,0.1028,4.9289,0f000001,0*b9d8443c\n\t", "INSPVAXA,USB3,0,51.0,FINESTEERING,2107,282991.150,02000000,471d,15824;INS_ALIGNMENT_COMPLETE,INS_RTKFIXED,37.37102077697,126.72358217095,8.4272,22.3000,0.1498,-0.2404,-0.0111,-0.329986353,-0.737306515,294.974204977,0.4460,0.2950,0.5595,0.1141,0.0925,0.0776,0.0977,0.1028,4.9303,0f000001,0*44f52417\n\t", "INSPVAXA,USB3,0,52.0,FINESTEERING,2107,282992.150,02000000,471d,15824;INS_ALIGNMENT_COMPLETE,INS_RTKFIXED,37.37102208780,126.72357933244,8.4219,22.3000,0.1505,-0.2512,-0.0006,-0.471923349,-0.884947239,294.718584068,0.4460,0.2949,0.5594,0.1141,0.0926,0.0776,0.0977,0.1028,4.9317,0f000001,0*525866c6\n\t", "INSPVAXA,USB3,0,42.5,FINESTEERING,2107,283000.150,02008000,471d,15824;INS_ALIGNMENT_COMPLETE,INS_RTKFIXED,37.37103215127,126.72355655993,8.3901,22.3000,0.1524,-0.2449,-0.0003,-0.362652962,-1.080137119,293.057786334,0.4445,0.2951,0.5592,0.1140,0.0926,0.0776,0.0977,0.1028,4.9425,0f000001,0*4235a1eb\n\t", "INSPVAXA,USB3,0,49.0,FINESTEERING,2107,283003.650,02008000,
